vi "testGalvoRamps.vi"() -> ()   [LabVIEW 2010]
panel:
  out "Galvo Ramps":dynamicdata(graph)
  out "Ramps_EnableRecording":T1
  out "Single ramps":dynamicdata(graph)
  out "Whole ramps":dynamicdata(graph)
  out "Volume recording done\nEnable recording":bool[][](array[boolean])
  out "samplesPerVolume":u32
  in  "Volume Dimensions":T2={"A-lines per B-frame"=512, "B-frames per volume"=50, "FOV (mm)"={"X"=10.0, "Y"=15.0}, "Scan type"=enum."Scan along X"}
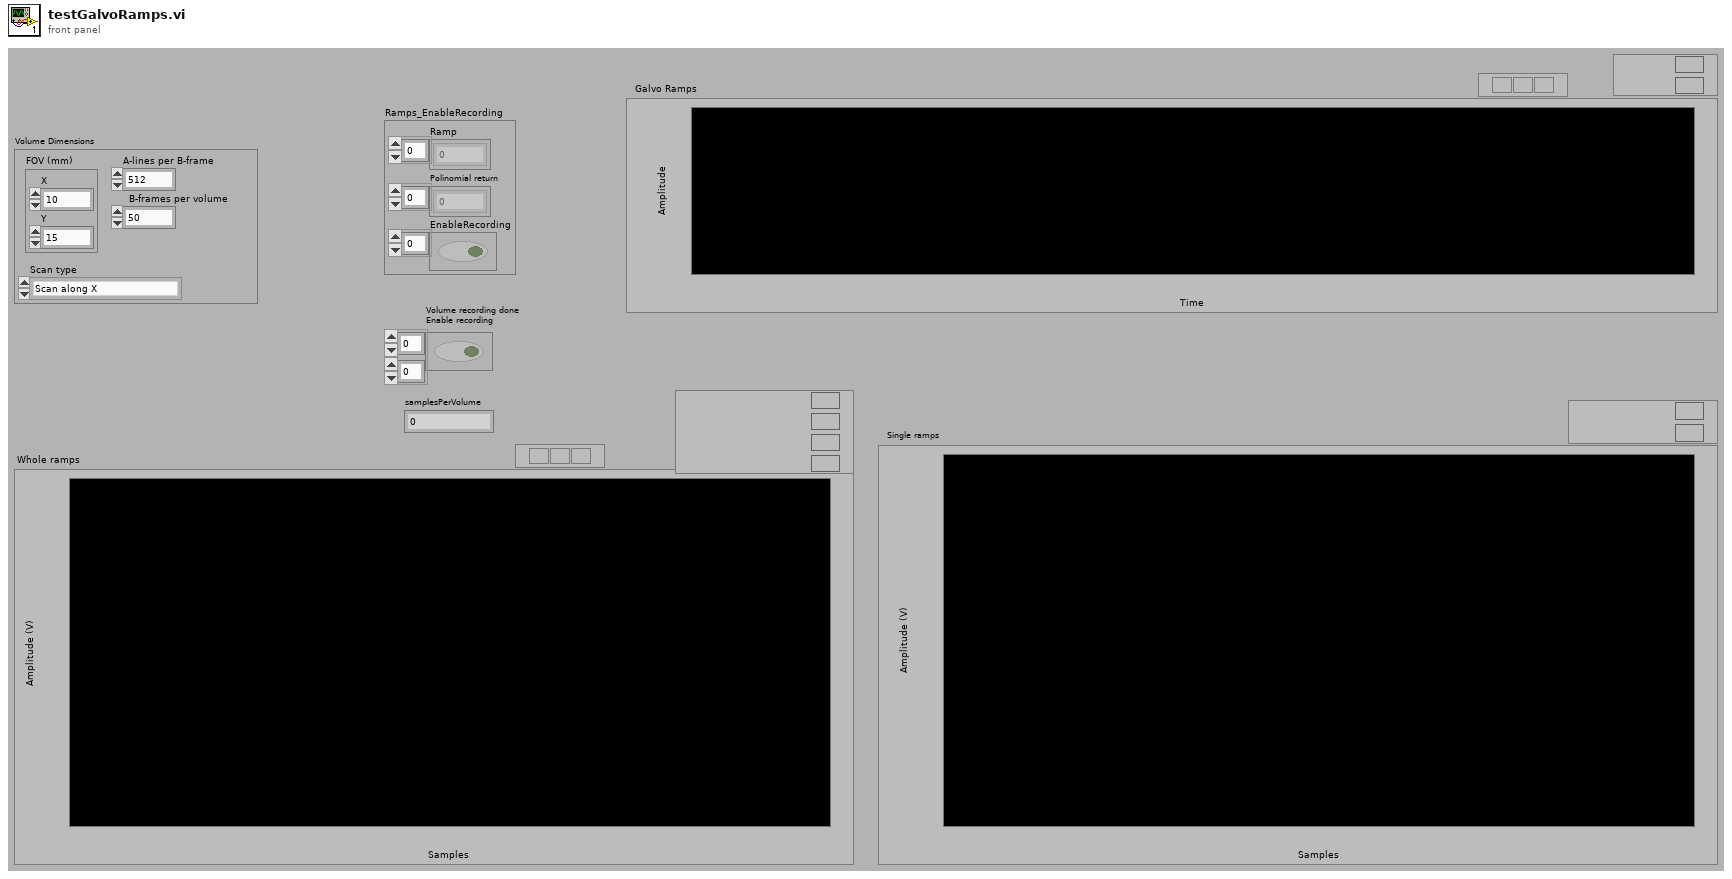
[diagram p1: front panel]
types:
  T1 = cluster{"Ramp":dbl[], "Polinomial return":dbl[], "EnableRecording":bool[]}
  T2 = cluster{"A-lines per B-frame":u16, "B-frames per volume":u16, "FOV (mm)":cluster{"X":dbl, "Y":dbl}, "Scan type":enum16{"Scan along X", "Scan along Y", "3D (Reverse Scan)"}}
  T3 = cluster{"X Start ":dbl, "X End ":dbl, "Y Start ":dbl, "Y End ":dbl}
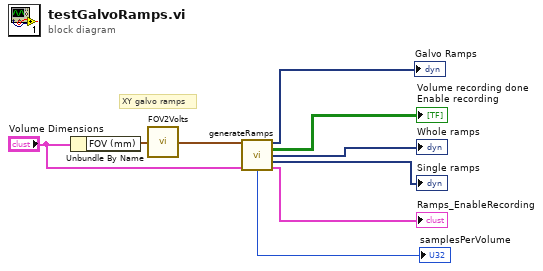
[diagram p0: block diagram]
diagram:
  # "XY galvo ramps"
  n1 = Unbundle By Name("Volume Dimensions") -> ("FOV (mm)"=w9:cluster{"X":dbl, "Y":dbl})
  n2 = call "FOV2Volts.vi"("FOV (mm)"=w9) -> ("VoltageGalvo"=w8:T3)
  n3 = call "generateRamps.vi"("Galvo Voltage"=w8, "Volume Dimensions"="Volume Dimensions") -> ("Galvo Ramps"=→"Galvo Ramps":dynamicdata, "Volume recording done\nEnable recording"=→"Volume recording done\nEnable recording":bool[][], "Whole ramps"=→"Whole ramps":dynamicdata, "Single ramps"=→"Single ramps":dynamicdata, "samplesPerVolume"=→"samplesPerVolume":u64, "Ramps_EnableRecording"=→"Ramps_EnableRecording":T1)  [unwired: 8 in]
